vi "_EnumEditor_BuildNewElementName.vi"(11 "ActualStrings":string[](array[string])) -> (3 "New string":string)   [LabVIEW 2014, in "_EnumEditor.lvclass"]
uses:
  _EnumEditor.lvclass
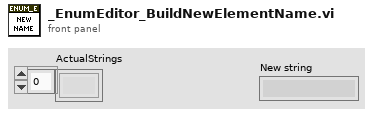
[diagram p1: front panel]
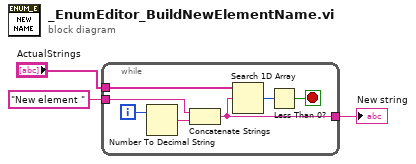
[diagram p0: block diagram]
diagram:
  n1 = while {
    tunnel: "ActualStrings" -> [w10]
    tunnel: "New element " -> [w8]
    tunnel: [w4] -> w3
    i -> [w9]
    stop <- w5 stop-if-true
    n2 = Number To Decimal String(number=w9) -> (decimal integer string=w7:string)  [unwired: 1 in]
    n3 = Concatenate Strings(w8, w7) -> (w4:string)
    n4 = Search 1D Array(1D array=w10, element=w4) -> (index of element=w6:i32)  [unwired: 1 in]
    n5 = Less Than 0?(x=w6) -> (x < 0?=w5:bool)
  }
  "New string" <- w3
